vi "Config and Read.vi"() -> ()   [LabVIEW 2020]
uses:
  DMM.NI/NI.Simulate/DMM.NI.Simulate.lvclass
  PPL/HDH.Driver.DMM.lvlibp/DMM Driver.lvclass
  PPL/HDH.Actor Framework.Core.Instrument Driver.lvlibp/Instrument Driver/Instrument Driver.lvclass
  C:/Current projects/WS/LV32.2020.HDH.Driver.DMM/DMM.NI/NI/DMM.NI.lvclass
  C:/Current projects/WS/PPL/HDH.Driver.DMM.lvlibp/DMM Driver.lvclass
  C:/Current projects/WS/PPL/HDH.Actor Framework.Core.Instrument Driver.lvlibp/Instrument Driver/Instrument Driver.lvclass
  PPL/HDH.Driver.DMM.lvlibp/Controls/Ctl_DigitResolution.ctl
  PPL/HDH.Driver.DMM.lvlibp
  PPL/HDH.Driver.DMM.lvlibp/Controls/Ctl_Function.ctl
panel:
  out "Digit Resolution read":T1=enum."5½"
  out "Range read":dbl
  out "Measurements":dbl[](array[numeric])
  out "Function read":T2
  in  "Measurements to Acquire(1)":i32=4 min=0
  in  "Max Time (-1ms)":i32=-1
  in  "Function":T2
  in  "Range":dbl=10.0
  in  "Digit Resolution(5½)":T1=enum."4½"
  out "Config Success?":bool
  out "error out":errorcluster
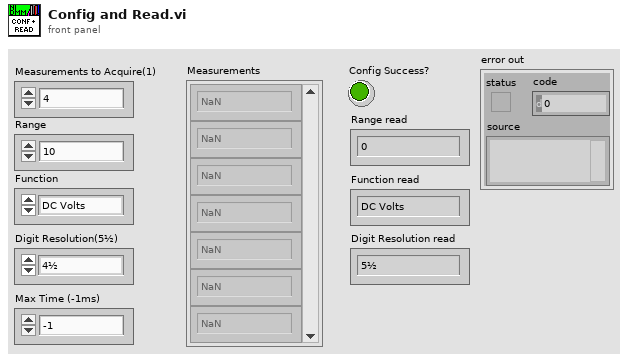
[diagram p1: front panel]
types:
  T1 = typedef "HDH.Driver.DMM.lvlibp/Ctl_DigitResolution.ctl" = enum8{"3½", "4½", "5½", "6½", "7½"}
  T2 = typedef "HDH.Driver.DMM.lvlibp/Ctl_Function.ctl" = enum8{"DC Volts", "AC Volts", "DC Current", "AC Current", "2-wire Resistance", "4-wire Resistance", "Diode", "Frequency", "Period", "AC Volts DC Coupled", "Capacitance", "Inductance", "Temperature"}
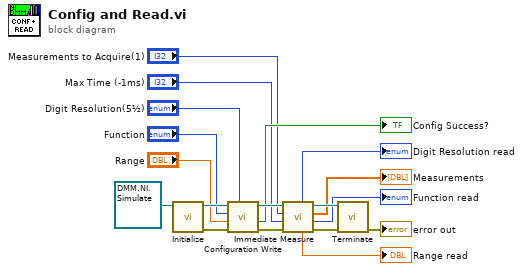
[diagram p0: block diagram]
diagram:
  n1 = call "Initialize.vi"("Instrument in"=refnum<class "DMM.NI.Simulate.lvclass"> refnum ("NI DMM Driver.lvlib:NI DMM Simulation Driver.lvclass")) -> ("error out"=w16:errorcluster, "Instrument out"=w17:refnum<class "DMM.NI.Simulate.lvclass">)  [unwired: 9 in]
  n2 = call "Configuration Write.vi"("Digit Resolution(5½)"="Digit Resolution(5½)", "error in (no error)"=w16, "Range"="Range", "Function"="Function", "DMM Driver in"=w17) -> ("error out"=w14:errorcluster, "Success?"=→"Config Success?":bool, "DMM Driver out"=w15:refnum<class "DMM.NI.Simulate.lvclass">)  [unwired: 4 in]
  n3 = call "Immediate Measure.vi"("error in (no error)"=w14, "Max Time (-1ms)"="Max Time (-1ms)", "Measurements to Acquire(1)"="Measurements to Acquire(1)", "DMM Driver in"=w15) -> ("error out"=w12:errorcluster, "Function"=→"Function read":T2, "Measurements"=→"Measurements":dbl[], "DMM Driver out"=w13:refnum<class "DMM.NI.Simulate.lvclass">, "Range"=→"Range read":dbl, "Digit Resolution(5½)"=→"Digit Resolution read":T1)  [unwired: 2 in]
  n4 = call-dynamic "Terminate.vi"("error in (no error)"=w12, "Instrument in"=w13) -> ("error out"=→"error out":errorcluster)  [unwired: 8 in, 1 out]
